vi "GFGnumericGet.vi"(7 "GFG Refnum (use when calling from external project)":refnum<vi>, 8 "error in (no error)":errorcluster, 11 "Variable Name in":string) -> (0 "error out":errorcluster, 3 "Numeric":dbl)   [LabVIEW 2012, in "GFG library.lvlib"]
uses:
  GFG library.lvlib
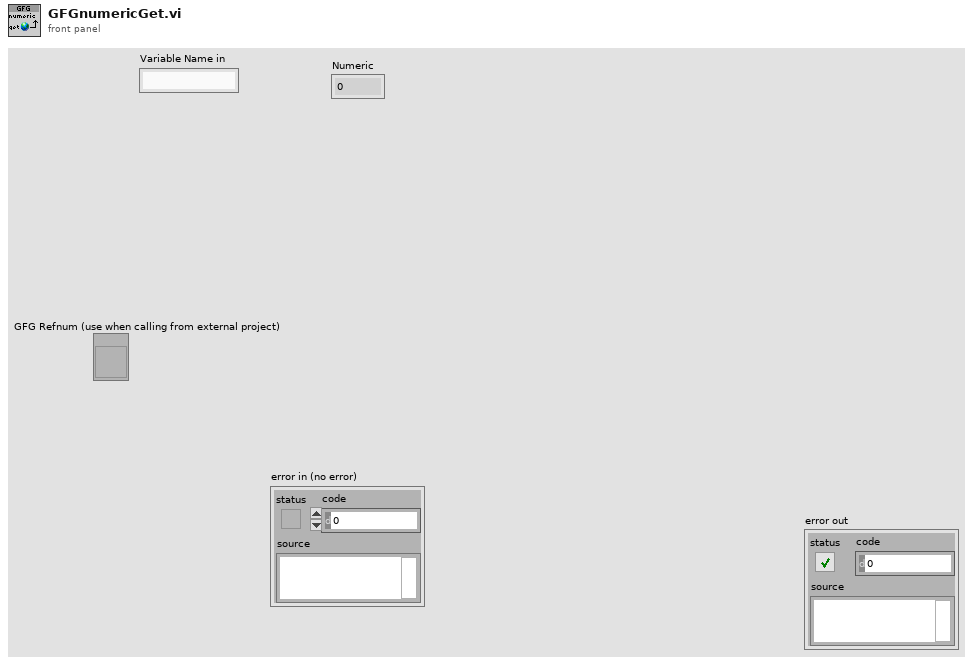
[diagram p1: front panel]
types:
  T1 = typedef "VariantType.lvlib/Type.ctl" = enum8{"Invalid Type", "Void", "I8", "I16", "I32", "I64", "U8", "U16", "U32", "U64", "Single Float", "Double Float", "Extended Float", "Single Complex", "Double Complex", "Extended Complex", "Enum U8", "Enum U16", "Enum U32", "Enum U64", "Single Float With Unit", "Double Float With Unit", "Extended Float With Unit", "Single Complex with Unit", "Double Complex with Unit", "Extended Complex with Unit", "Boolean", "String", "Path", "Picture", "Tag", "Array", "Cluster", "Variant", "LV Variant", "Waveform", "Timestamp", "Digital Waveform", "Digital Data", "ExpressData", "Refnum", "External Data", "VI", "Poly VI", "LabVIEW Class Instance", "Fixed Point"}
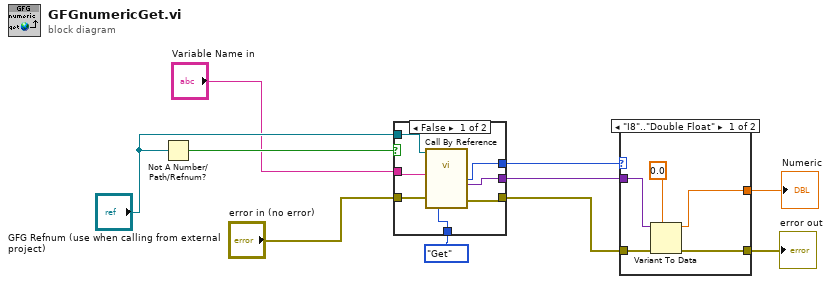
[diagram p0: block diagram]
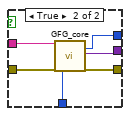
[diagram p2: hidden frame]
diagram:
  n1 = Not A Number/Path/Refnum?(number/path/refnum="GFG Refnum (use when calling from external project)") -> (NaN/Path/Refnum?=w6:bool)
  n2 = case shown="False" w6 {
    tunnel: enum16{"Init", "Set", "Get"}."Get" ("Action") -> [w12 w23]
    tunnel: "Variable Name in" -> [w13 w22]
    tunnel: "error in (no error)" -> [w17 w21]
    tunnel: [w16 w20] -> w3
    tunnel: [w14 w19] -> w1
    tunnel: [w15 w18] -> w2
    tunnel: "GFG Refnum (use when calling from external project)" -> [w11 _]
    frame False {
      n3 = call-by-ref "?"(reference=w11, "Variable Name in"=w13, "error in (no error)"=w17, "Action"=w12) -> ("Data Type Out"=w14:T1, "Variant Out"=w15:variant, "error out"=w16:errorcluster)  [unwired: 11 in, 6 out]
    }
    frame True {
      n4 = call "GFG_core.vi"("Variable Name in"=w22, "error in (no error)"=w21, "Action"=w23) -> ("Data Type Out"=w19:T1, "Variant Out"=w18:variant, "error out"=w20:errorcluster)  [unwired: 10 in, 4 out]
    }
  }
  n5 = case shown="\"I8\"..\"Double Float\"" w1 {
    tunnel: w2 -> [w27 _]
    tunnel: [w26 _] -> w10
    tunnel: [w24 w29] -> w9
    tunnel: w3 -> [w25 w29]
    frame "I8".."Double Float" {
      n6 = Variant To Data(error in=w25, type=0.0, Variant=w27) -> (data=w26:dbl, error out=w24:errorcluster)
    }
    frame Default {
    }
  }
  "Numeric" <- w10
  "error out" <- w9
